vi "GetName.vi"(8 "Error In":errorcluster, 11 "object in":refnum<class "YAFTAF.lvclass">) -> (0 "Error Out":errorcluster, 2 "Name":string, 3 "object out":refnum<class "YAFTAF.lvclass">)   [LabVIEW 2021, in "YAFTAF.lvclass"]
uses:
  YAFTAF.lvclass
  C:/Localdata/Projects/TriekselSoft/TriekselsoftApplicationFramework/Source/.Externals/Library_YAF/YActor/YActor.lvclass
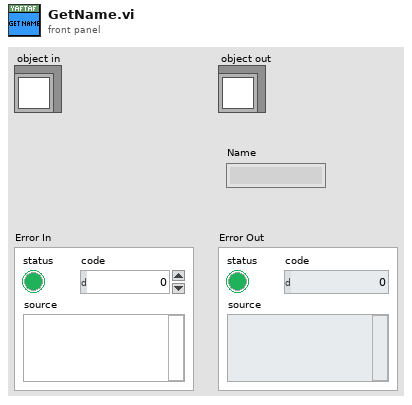
[diagram p1: front panel]
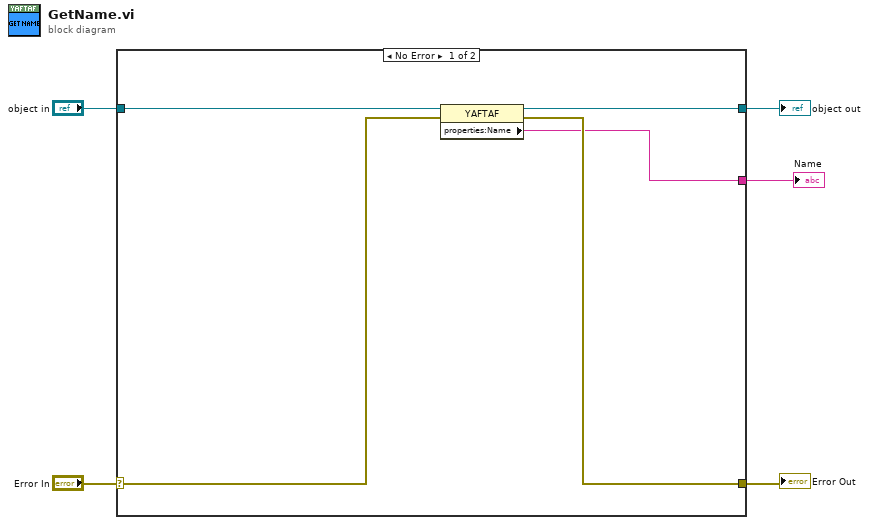
[diagram p0: block diagram]
diagram:
  n1 = case shown="No Error" "Error In" {
    selector: "Error In" -> [w8 w12]
    tunnel: [w7 w12] -> w4
    tunnel: [w9 w11] -> w2
    tunnel: "object in" -> [w10 w11]
    tunnel: [w6 _] -> w1
    frame No Error {
      n2 = property class="YAFTAF"(reference=w10, error in=w8) -> (reference out=w9:refnum<class "YAFTAF.lvclass">, error out=w7:errorcluster, "properties:Name"=w6:string)
    }
    frame Error {
    }
  }
  "Error Out" <- w4
  "object out" <- w2
  "Name" <- w1
